vi "JKI SM Core - Post-Build Custom Action.vi"(10 "Variant":variant) -> (0 "error out":errorcluster)   [LabVIEW 2013]
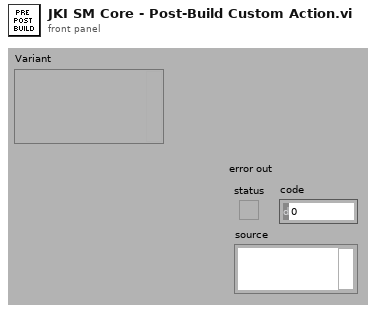
[diagram p1: front panel]
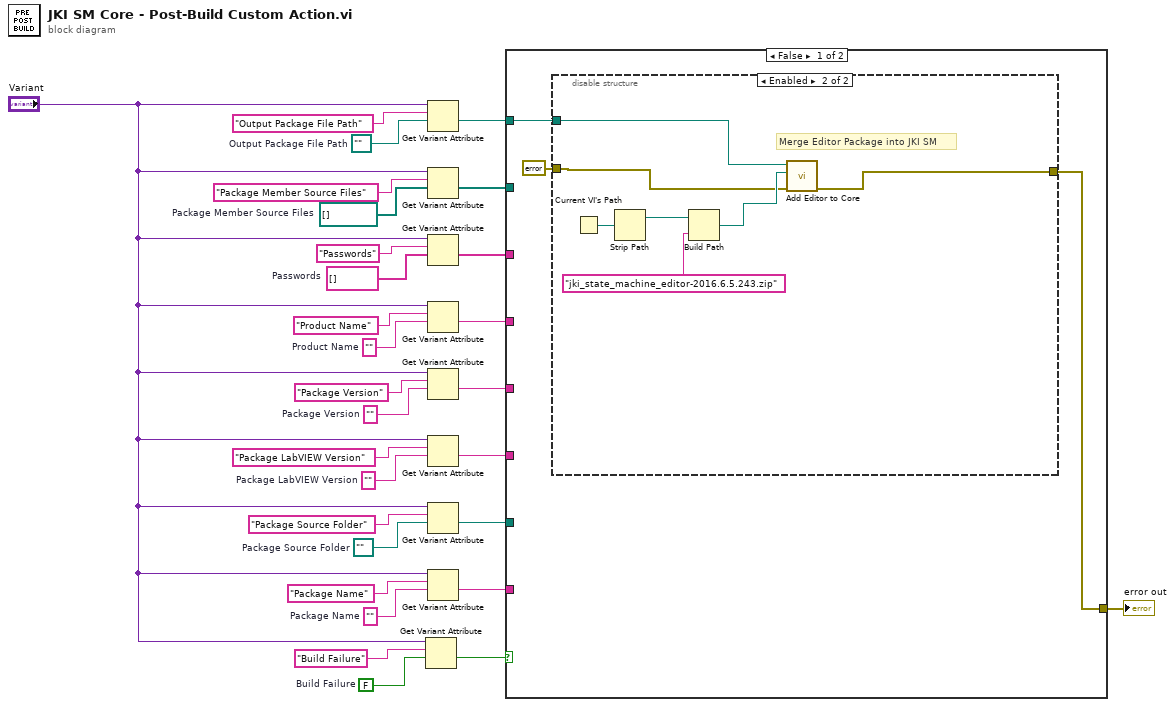
[diagram p0: block diagram]
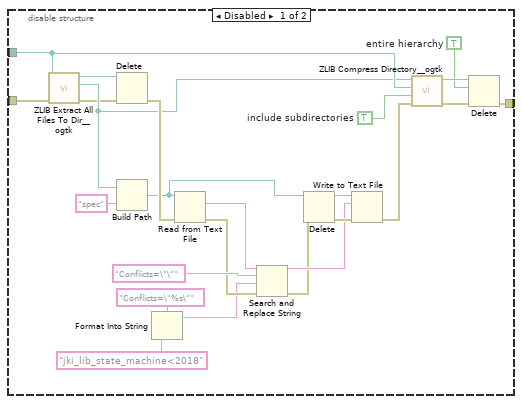
[diagram p2: hidden frame]
diagram:
  w4 = FALSE  # Build Failure
  w14 = path ""  # Package Source Folder
  w15 = ""  # Package Name
  w18 = ""  # Package LabVIEW Version
  w20 = ""  # Package Version
  w22 = ""  # Product Name
  w24 = string[] []  # Passwords
  w26 = path[] []  # Package Member Source Files
  w28 = path ""  # Output Package File Path
  n1 = Get Variant Attribute(Variant="Variant", name="Build Failure", default value (empty Variant)=w4) -> (value=w1:bool)  [unwired: 1 in, 3 out]
  n2 = Get Variant Attribute(Variant="Variant", name="Output Package File Path", default value (empty Variant)=w28) -> (value=w13:path)  [unwired: 1 in, 3 out]
  n3 = Get Variant Attribute(Variant="Variant", name="Package Member Source Files", default value (empty Variant)=w26) -> (value=w12:path[])  [unwired: 1 in, 3 out]
  n4 = Get Variant Attribute(Variant="Variant", name="Passwords", default value (empty Variant)=w24) -> (value=w11:string[])  [unwired: 1 in, 3 out]
  n5 = Get Variant Attribute(Variant="Variant", name="Product Name", default value (empty Variant)=w22) -> (value=w10:string)  [unwired: 1 in, 3 out]
  n6 = Get Variant Attribute(Variant="Variant", name="Package Version", default value (empty Variant)=w20) -> (value=w9:string)  [unwired: 1 in, 3 out]
  n7 = Get Variant Attribute(Variant="Variant", name="Package LabVIEW Version", default value (empty Variant)=w18) -> (value=w8:string)  [unwired: 1 in, 3 out]
  n8 = Get Variant Attribute(Variant="Variant", name="Package Source Folder", default value (empty Variant)=w14) -> (value=w7:path)  [unwired: 1 in, 3 out]
  n9 = Get Variant Attribute(Variant="Variant", name="Package Name", default value (empty Variant)=w15) -> (value=w6:string)  [unwired: 1 in, 3 out]
  n10 = case shown="False" w1 {
    tunnel: w13 -> [w32 _]
    tunnel: w12 -> [_ _]
    tunnel: w11 -> [_ _]
    tunnel: w10 -> [_ _]
    tunnel: w9 -> [_ _]
    tunnel: w8 -> [_ _]
    tunnel: w7 -> [_ _]
    tunnel: w6 -> [_ _]
    tunnel: [w31 _] -> w2
    frame False {
      n11 = disable-structure shown="Enabled" {
        disable-tunnel: w32 -> [w56 w63]
        disable-tunnel: [w55 w59] -> w31
        disable-tunnel: errorcluster {"status"=FALSE, "code"=0, "source"=""} ("error in (no error)") -> [w54 w60]
        frame Disabled {
          w39 = TRUE  # include subdirectories
          w51 = TRUE  # entire hierarchy
          n12 = call <userlib>:"ZLIB Extract All Files To Dir__ogtk.vi"("error in (no error)"=w54, "archive name (file dialog)"=w56) -> ("error out"=w36:errorcluster, "root directory out"=w38:path, "archive name out"=w37:path)  [unwired: 7 in]
          n13 = Delete(path (use dialog)=w37, error in=w36) -> (error out=w46:errorcluster)  [unwired: 3 in, 2 out]
          n14 = Build Path(base path=w38, name or relative path="spec") -> (appended path=w45:path)
          n15 = Format Into String(format string="Conflicts=\"%s\"" ("search string"), "jki_lib_state_machine<2018" ("search string")) -> (resulting string=w35:string)  [unwired: 2 in, 1 out]
          n16 = Read from Text File(file (use dialog)=w45, error in=w46) -> (text=w49:string, error out=w47:errorcluster)  [unwired: 2 in, 2 out]
          n17 = Search and Replace String(input string=w49, search string="Conflicts=\"\"", replace string=w35, error in=w47) -> (result string=w42:string, error out=w41:errorcluster)  [unwired: 4 in, 2 out]
          n18 = Delete(path (use dialog)=w45, error in=w41) -> (deleted path=w43:path, error out=w44:errorcluster)  [unwired: 3 in, 1 out]
          n19 = Write to Text File(file (use dialog)=w43, text=w42, error in=w44) -> (error out=w40:errorcluster)  [unwired: 1 in, 2 out]
          n20 = call <userlib>:"ZLIB Compress Directory__ogtk.vi"("error in (no error)"=w40, "include subdirectories (F)"=w39, "archive name (root directory with .zip ending)"=w56, "root directory (file dialog)"=w38) -> ("error out"=w53:errorcluster, "root directory out"=w52:path)  [unwired: 5 in, 1 out]
          n21 = Delete(path (use dialog)=w52, entire hierarchy (F)=w51, error in=w53) -> (error out=w55:errorcluster)  [unwired: 2 in, 2 out]
        }
        frame Enabled {
          # "Merge Editor Package into JKI SM"
          n22 = Current VI's Path() -> (path=w58:path)
          n23 = Strip Path(path=w58) -> (stripped path=w57:path)  [unwired: 1 out]
          n24 = Build Path(base path=w57, name or relative path="jki_state_machine_editor-2016.6.5.243.zip") -> (appended path=w61:path)
          n25 = call "Add Editor to Core.vi"("error in (no error)"=w60, "JKI State Machine Editor Package"=w61, "JKI State Machine Package"=w63) -> ("error out"=w59:errorcluster)  [unwired: 8 in]
        }
      }
    }
    frame True {
    }
  }
  "error out" <- w2
